vi "form alarm string.vi"(0 "Vmon":dbl[][](array[numeric]), 1 "Vset":dbl[][](array[numeric]), 2 "Imon":dbl[][](array[numeric]), 3 "Iset":dbl[][](array[numeric]), 4 "Timestamps":dbl[][](array[numeric]), 5 "error in":errorcluster, 8 "Start index":i32, 9 "Crate":i32, 10 "Num Channels Read":i32) -> (14 "Alarm String":string, 15 "Background colour":u32, 16 "All alarms string":string, 17 "Alarm Array":string[][](array[string]), 18 "Alarm":bool, 19 "error out":errorcluster)   [LabVIEW 2018]
uses:
  CAEN globals.vi
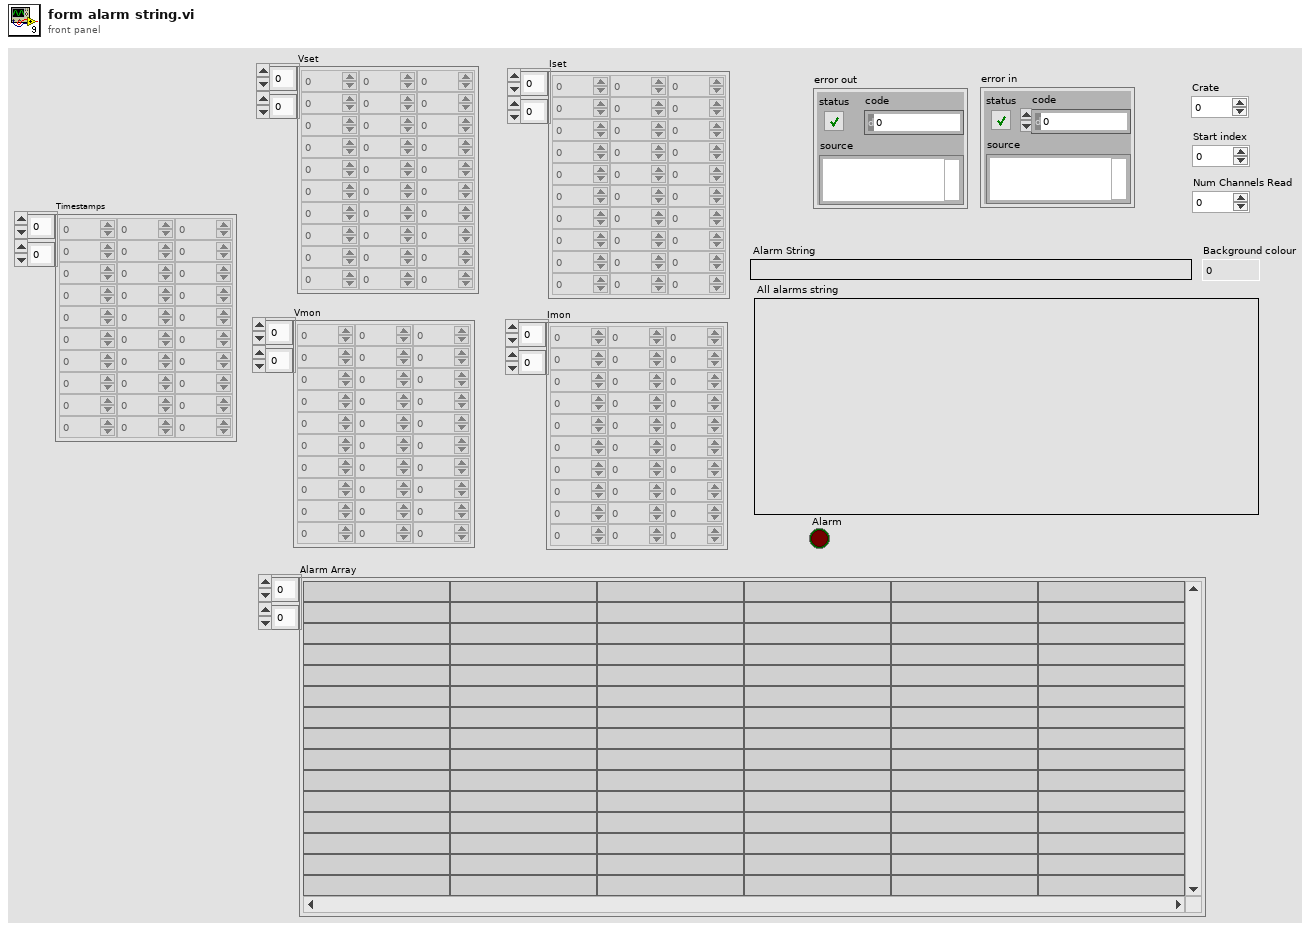
[diagram p1: front panel]
types:
  T1 = typedef "channel_cluster.ctl" = cluster{"Channel Name":string, "Crate":i32, "Card Type":string, "Card":i32, "Channel":i32, "Status Icon":picture, "Vmon (V)":dbl, "Vset (V)":dbl, "Imon (A)":dbl, "Iset (A)":dbl, "Timestamp":string, "ON/OFF":bool, "Status":string, "Vswmax (V)":dbl, "Flag":bool, "Vfile (V)":dbl, "Error Logged":bool[], "enable_file":bool}
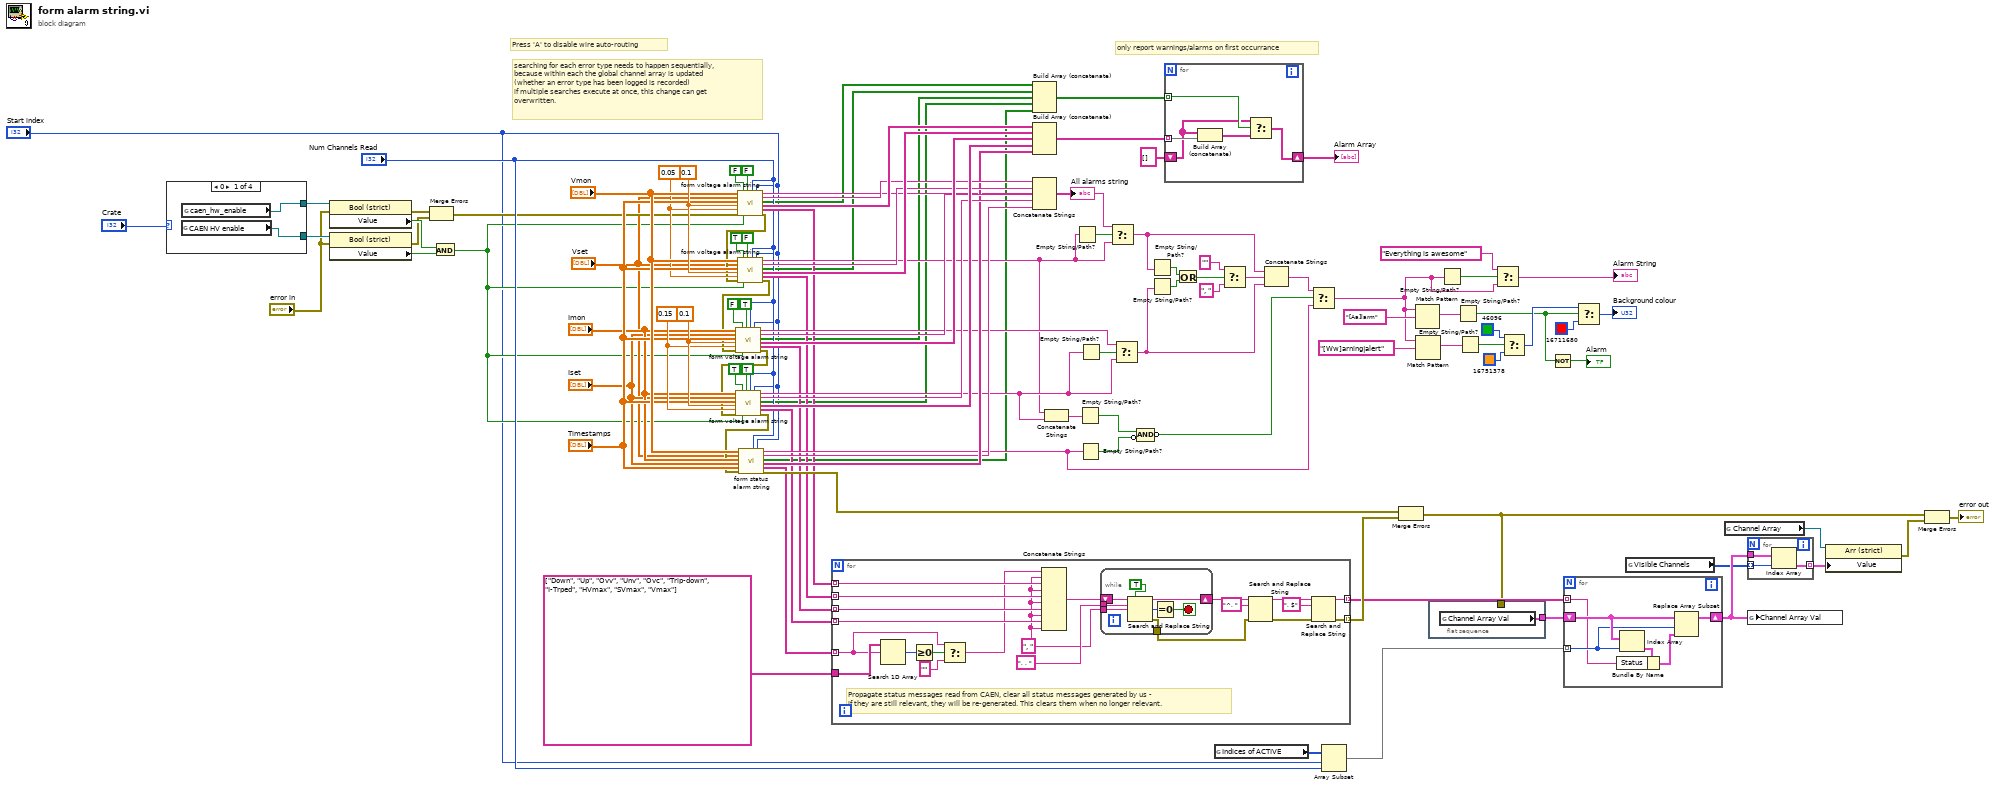
[diagram p0: block diagram]
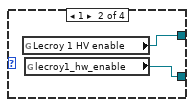
[diagram p2: hidden frame]
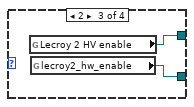
[diagram p3: hidden frame]
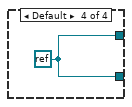
[diagram p4: hidden frame]
diagram:
  w67 = 0.15 ("Tolerance (%)")
  w68 = 0.1 ("Tolerance (%)")
  w19 = 0.05 ("Tolerance (%)")
  w69 = 0.1 ("Tolerance (%)")
  # "Press 'A' to disable wire auto-routing"
  # "searching for each error type needs to happen sequentially,\nbecause within each the global channel array is updated\n(whether an error type has been logged is recorded)\nif multiple searches execute at once, this change can get\noverwritten."
  # "only report warnings/alarms on first occurrance"
  n1 = case shown="0" "Crate" {
    tunnel: [w110 w112 w114 w115] -> w7
    tunnel: [w109 w111 w113 w115] -> w6
    frame 0 {
      n2 = global read "CAEN globals.vi" "CAEN HV enable"() -> (w109:refnum<vi>)
      n3 = global read "CAEN globals.vi" "caen_hw_enable"() -> (w110:refnum<vi>)
    }
    frame 1 {
      n4 = global read "CAEN globals.vi" "Lecroy 1 HV enable"() -> (w112:refnum<vi>)
      n5 = global read "CAEN globals.vi" "lecroy1_hw_enable"() -> (w111:refnum<vi>)
    }
    frame 2 {
      n6 = global read "CAEN globals.vi" "Lecroy 2 HV enable"() -> (w114:refnum<vi>)
      n7 = global read "CAEN globals.vi" "lecroy2_hw_enable"() -> (w113:refnum<vi>)
    }
    frame Default {
      w115 = refnum<k0> refnum
    }
  }
  n8 = property class="Bool (strict)"(reference=w7, error in="error in") -> (error out=w8:errorcluster, "Value"=w10:bool)  [unwired: 1 out]
  n9 = property class="Bool (strict)"(reference=w6, error in="error in") -> (error out=w9:errorcluster, "Value"=w11:bool)  [unwired: 1 out]
  n10 = Merge Errors(w8, w9) -> (w12:errorcluster)
  n11 = And(x=w10, y=w11) -> (x .and. y?=w4:bool)
  n12 = call "form voltage alarm string.vi"("Xmon"="Vmon", "Xset"="Vset", "Timestamps"="Timestamps", "Alarm Tolerance (frac)"=w69, "Warning Tolerance (frac)"=w19, "error in"=w12, "Alarm:T Warning:F"=FALSE ("Current:T Voltage:F"), "Crate Enable"=w4, "Current:T Voltage:F"=FALSE, "Num Channels Read"="Num Channels Read", "Start index"="Start index") -> ("Error Status String"=w59:string, "All channels in error"=w79:string, "Error Logged"=w27:bool[], "Error Array"=w88:string[][], "Status Strings"=w45:string[], "Error Out"=w18:errorcluster)  [unwired: 3 in]
  n13 = call "form voltage alarm string.vi"("Xmon"="Vmon", "Xset"="Vset", "Timestamps"="Timestamps", "Alarm Tolerance (frac)"=w69, "Warning Tolerance (frac)"=w19, "error in"=w18, "Alarm:T Warning:F"=TRUE ("Current:T Voltage:F"), "Crate Enable"=w4, "Current:T Voltage:F"=FALSE, "Num Channels Read"="Num Channels Read", "Start index"="Start index") -> ("Error Status String"=w49:string, "All channels in error"=w80:string, "Error Logged"=w28:bool[], "Error Array"=w87:string[][], "Status Strings"=w44:string[], "Error Out"=w17:errorcluster)  [unwired: 3 in]
  n14 = call "form voltage alarm string.vi"("Xmon"="Imon", "Xset"="Iset", "Timestamps"="Timestamps", "Alarm Tolerance (frac)"=w68, "Warning Tolerance (frac)"=w67, "error in"=w17, "Alarm:T Warning:F"=FALSE ("Current:T Voltage:F"), "Crate Enable"=w4, "Current:T Voltage:F"=TRUE, "Num Channels Read"="Num Channels Read", "Start index"="Start index") -> ("Error Status String"=w58:string, "All channels in error"=w81:string, "Error Logged"=w26:bool[], "Error Array"=w85:string[][], "Status Strings"=w43:string[], "Error Out"=w16:errorcluster)  [unwired: 3 in]
  n15 = call "form voltage alarm string.vi"("Xmon"="Imon", "Xset"="Iset", "Timestamps"="Timestamps", "Alarm Tolerance (frac)"=w68, "Warning Tolerance (frac)"=w67, "error in"=w16, "Alarm:T Warning:F"=TRUE ("Current:T Voltage:F"), "Crate Enable"=w4, "Current:T Voltage:F"=TRUE, "Num Channels Read"="Num Channels Read", "Start index"="Start index") -> ("Error Status String"=w50:string, "All channels in error"=w82:string, "Error Logged"=w25:bool[], "Error Array"=w86:string[][], "Status Strings"=w42:string[], "Error Out"=w15:errorcluster)  [unwired: 3 in]
  n16 = call "form status alarm string.vi"("Vmon"="Vmon", "Vset"="Vset", "Imon"="Imon", "Iset"="Iset", "Timestamps"="Timestamps", "error in"=w15, "Num Channels Read"="Num Channels Read", "Start index"="Start index") -> ("Error Status String"=w53:string, "All channels in error"=w60:string, "Error Logged"=w24:bool[], "Error Array"=w61:string[][], "Status Strings"=w41:string[], "Error Out"=w62:errorcluster)  [unwired: 6 in]
  n17 = for {
    tunnel: w45 -> [w136] mode=indexing
    tunnel: w44 -> [w135] mode=indexing
    tunnel: w43 -> [w134] mode=indexing
    tunnel: w42 -> [w133] mode=indexing
    tunnel: w41 -> [w118] mode=indexing
    tunnel: [w125] -> w34 mode=indexing
    tunnel: [w123] -> w40 mode=indexing
    tunnel: string[] ["Down", "Up", "Ovv", "Unv", "Ovc", "Trip-down", "I-Trped", "HVmax", "SVmax", "Vmax"] -> [w121]
    w126 = ", " ("Error Status String")
    # "Propagate status messages read from CAEN, clear all status messages generated by us - \nif they are still relevant, they will be re-generated. This clears them when no longer relevant."
    n18 = Search 1D Array(1D array=w121, element=w118) -> (index of element=w120:i32)  [unwired: 1 in]
    n19 = Greater Or Equal To 0?(x=w120) -> (x >= 0?=w119:bool)
    n20 = Select(t=w118, s=w119, f="") -> (s? t:f=w116:string)
    n21 = Concatenate Strings(w116, w126, w136, w126, w135, w126, w134, w126, w133, w126) -> (w128:string)
    n22 = while {
      tunnel: ", , " ("Error Status String") -> [w144]
      tunnel: w126 -> [w143]
      shift-right: [w142] -> w132
      shift-left: w128 -> [w141]
      tunnel: [w137] -> w122
      stop <- w138 stop-if-true
      n23 = Search and Replace String(replace all?=TRUE ("replace all? (F)"), input string=w141, search string=w144, replace string=w143) -> (result string=w142:string, number of replacements=w139:i32, error out=w137:errorcluster)  [unwired: 4 in, 1 out]
      n24 = Equal To 0?(x=w139) -> (x = 0?=w138:bool)
    }
    n25 = Search and Replace String(input string=w132, search string="^, ", error in=w122) -> (result string=w131:string, error out=w124:errorcluster)  [unwired: 5 in, 2 out]
    n26 = Search and Replace String(input string=w131, search string=", $", error in=w124) -> (result string=w125:string, error out=w123:errorcluster)  [unwired: 5 in, 2 out]
  }
  n27 = Build Array (concatenate)(w27, w28, w26, w25, w24) -> (w23:bool[])
  n28 = Build Array (concatenate)(w88, w87, w85, w86, w61) -> (w22:string[][])
  n29 = Concatenate Strings(w79, w80, w81, w82, w60) -> (→"All alarms string":string)
  n30 = Concatenate Strings(w49, w50) -> (w57:string)
  n31 = Empty String/Path?(string/path=w49) -> (empty?=w98:bool)
  n32 = Empty String/Path?(string/path=w57) -> (empty?=w56:bool)
  n33 = Empty String/Path?(string/path=w53) -> (empty?=w55:bool)
  n34 = Empty String/Path?(string/path=w50) -> (empty?=w97:bool)
  n35 = Select(t=w59, s=w98, f=w49) -> (s? t:f=w96:string)
  n36 = Select(t=w58, s=w97, f=w50) -> (s? t:f=w95:string)
  n37 = Compound Arithmetic op=AND(w56, invert w55) -> (invert w54:bool)
  n38 = Empty String/Path?(string/path=w96) -> (empty?=w94:bool)
  n39 = Empty String/Path?(string/path=w95) -> (empty?=w93:bool)
  n40 = for {
    tunnel: w23 -> [w148] mode=indexing
    tunnel: w22 -> [w149] mode=indexing
    shift-right: [w146] -> w20
    shift-left: string[][] [] ("appended array") -> [w145]
    n41 = Build Array (concatenate)(w145, w149) -> (w147:string[][])
    n42 = Select(t=w145, s=w148, f=w147) -> (s? t:f=w146:string[][])
  }
  "Alarm Array" <- w20
  n43 = Or(x=w94, y=w93) -> (x .or. y?=w92:bool)
  n44 = global read "CAEN globals.vi" "Indices of ACTIVE"() -> (w31:i32[])
  n45 = Select(t="" ("string"), s=w92, f=", " ("string")) -> (s? t:f=w89:string)
  n46 = Concatenate Strings(w96, w89, w95) -> (w52:string)
  n47 = Select(t=w52, s=w54, f=w53) -> (s? t:f=w51:string)
  n48 = Array Subset(array=w31, index="Start index", length="Num Channels Read") -> (w29:i32[])
  n49 = Merge Errors(w62, w40) -> (w13:errorcluster)
  n50 = Match Pattern(string=w51, regular expression="[Aa]larm") -> (match substring=w106:string)  [unwired: 1 in, 3 out]
  n51 = Match Pattern(string=w51, regular expression="[Ww]arning|alert") -> (match substring=w105:string)  [unwired: 1 in, 3 out]
  n52 = flat-sequence {
    tunnel: [w150] -> w14
    tunnel: w13 -> [_]
    frame #0 {
      n53 = global read "CAEN globals.vi" "Channel Array Val"() -> (w150:T1[])
    }
  }
  n54 = Empty String/Path?(string/path=w51) -> (empty?=w74:bool)
  n55 = Empty String/Path?(string/path=w106) -> (empty?=w70:bool)
  n56 = Empty String/Path?(string/path=w105) -> (empty?=w104:bool)
  n57 = Select(t="Everything is awesome" ("string"), s=w74, f=w51) -> (s? t:f=→"Alarm String":string)
  n58 = Select(t=u32 46096, s=w104, f=u32 16751378) -> (s? t:f=w101:u32)
  n59 = Not(x=w70) -> (.not. x?=→"Alarm":bool)
  n60 = for {
    shift-right: [w154] -> w38
    shift-left: w14 -> [w156]
    tunnel: w29 -> [w155] mode=indexing
    tunnel: w34 -> [w151] mode=indexing
    n61 = Index Array(array=w156, index=w155) -> (element=w153:T1)
    n62 = Bundle By Name(cluster=w153, "Status"=w151) -> (w152:T1)
    n63 = Replace Array Subset(array=w156, new element=w152, index=w155) -> (w154:T1[])
  }
  n64 = Select(t=w101, s=w70, f=u32 16711680) -> (s? t:f=→"Background colour":u32)
  n65 = global read "CAEN globals.vi" "Visible Channels"() -> (w37:i32[])
  n66 = global read "CAEN globals.vi" "Channel Array"() -> (w36:refnum<vi>)
  n67 = for {
    tunnel: w38 -> [w159]
    tunnel: w37 -> [w158] mode=indexing
    tunnel: [w157] -> w35 mode=indexing
    n68 = Index Array(array=w159, index=w158) -> (element=w157:T1)
  }
  n69 = global write "CAEN globals.vi" "Channel Array Val"(w38) -> ()
  n70 = property class="Arr (strict)"(reference=w36, "Value"=w35) -> (error out=w33:errorcluster)  [unwired: 1 in, 1 out]
  n71 = Merge Errors(w13, w33) -> (→"error out":errorcluster)
